vi "AddVIToClass.vi"(6 "Destination Folder":refnum<vi>, 7 "Access":T1, 8 "error in (no error)":errorcluster, 9 "Proposed VI Name":string, 10 "vi refnum in":refnum<vi>, 11 "LVClassLibrary Ref":refnum<vi>) -> (0 "error out":errorcluster, 1 "New project item ref":refnum<vi>, 2 "vi refnum out":refnum<vi>, 3 "LVClassLibrary Refnum out":refnum<vi>)   [LabVIEW 2021, in "MemberVICreation.lvlib" / "BaseAccessorScripter.lvclass"]
uses:
  <resource>/Framework/Providers/LVClassLibrary/NewAccessors/BaseAccessorScripter/BaseAccessorScripter.lvclass
  <resource>/Framework/Providers/LVClassLibrary/NewAccessors/CLSUIP_Access.ctl
  <resource>/Framework/Providers/LVClassLibrary/NewAccessors/MemberVICreation.lvlib
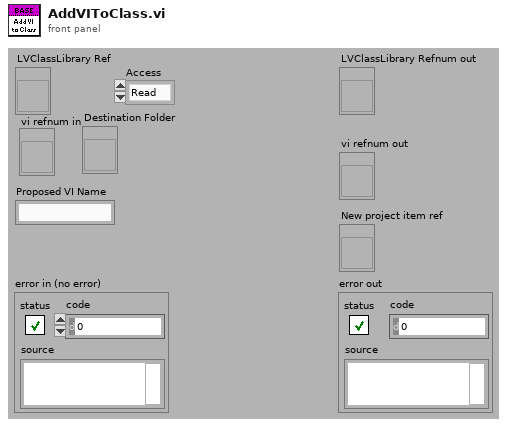
[diagram p1: front panel]
types:
  T1 = typedef "MemberVICreation.lvlib/CLSUIP_Access.ctl" = enum16{"Read", "Write", "R/W"}
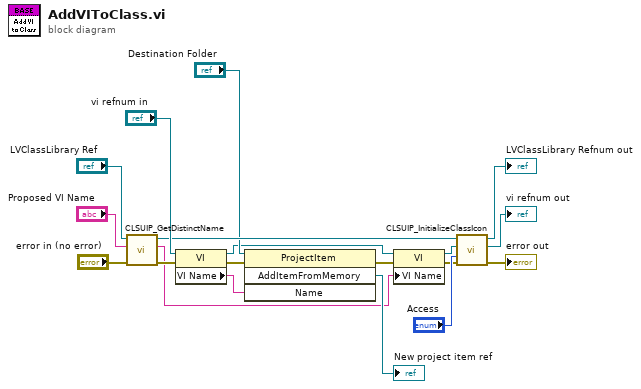
[diagram p0: block diagram]
diagram:
  n1 = call <resource>:"CLSUIP_GetDistinctName.vi"("error in (no error)"="error in (no error)", "Proposed name"="Proposed VI Name", "LVClassLibrary Refnum"="LVClassLibrary Ref") -> ("error out"=w19:errorcluster, "Accepted name"=w1:string, "LVClassLibrary Refnum out"=w10:refnum<vi>)  [unwired: 6 out]
  n2 = property class="VI"(reference="vi refnum in", error in=w19) -> (reference out=w3:refnum<vi>, error out=w9:errorcluster, "VI Name"=w6:string)
  n3 = invoke class="ProjectItem" method="AddItemFromMemory"(reference="Destination Folder", error in=w9, "Name"=w6) -> (error out=w5:errorcluster, "AddItemFromMemory"=→"New project item ref":refnum<vi>)  [unwired: 1 in, 2 out]
  n4 = property class="VI"(reference=w3, error in=w5, "VI Name"=w1) -> (reference out=w2:refnum<vi>, error out=w4:errorcluster)
  n5 = call <resource>:"CLSUIP_InitializeClassIcon.vi"("error in (no error)"=w4, "Access"="Access", "vi refnum in"=w2, "LVClassLibrary Refnum"=w10) -> ("error out"=→"error out":errorcluster, "vi refnum out"=→"vi refnum out":refnum<vi>, "LVClassLibrary Refnum out"=→"LVClassLibrary Refnum out":refnum<vi>)  [unwired: 5 out]
